vi "固件升级（包含参数恢复）.vi"() -> (3 "结果字符串":string)   [LabVIEW 2016, in "斯坦道总磷总氮.lvlib"]
uses:
  <vilib>/NI/Progress Bar/Controls/Progress Bar Properties.ctl
  <vilib>/Utility/error.llb/DialogType.ctl
  <vilib>/NI/Progress Bar/Progress Bar.lvlib
panel:
  out "布尔":bool
  out "仪器公式":T1(array[cluster])
  out "量程参数":T2(array[cluster])
  out "试剂容量参数":T3
  out "外设参数":cluster{"仪器版本":T4, "error out":errorcluster}
  out "固件升级步骤":T5
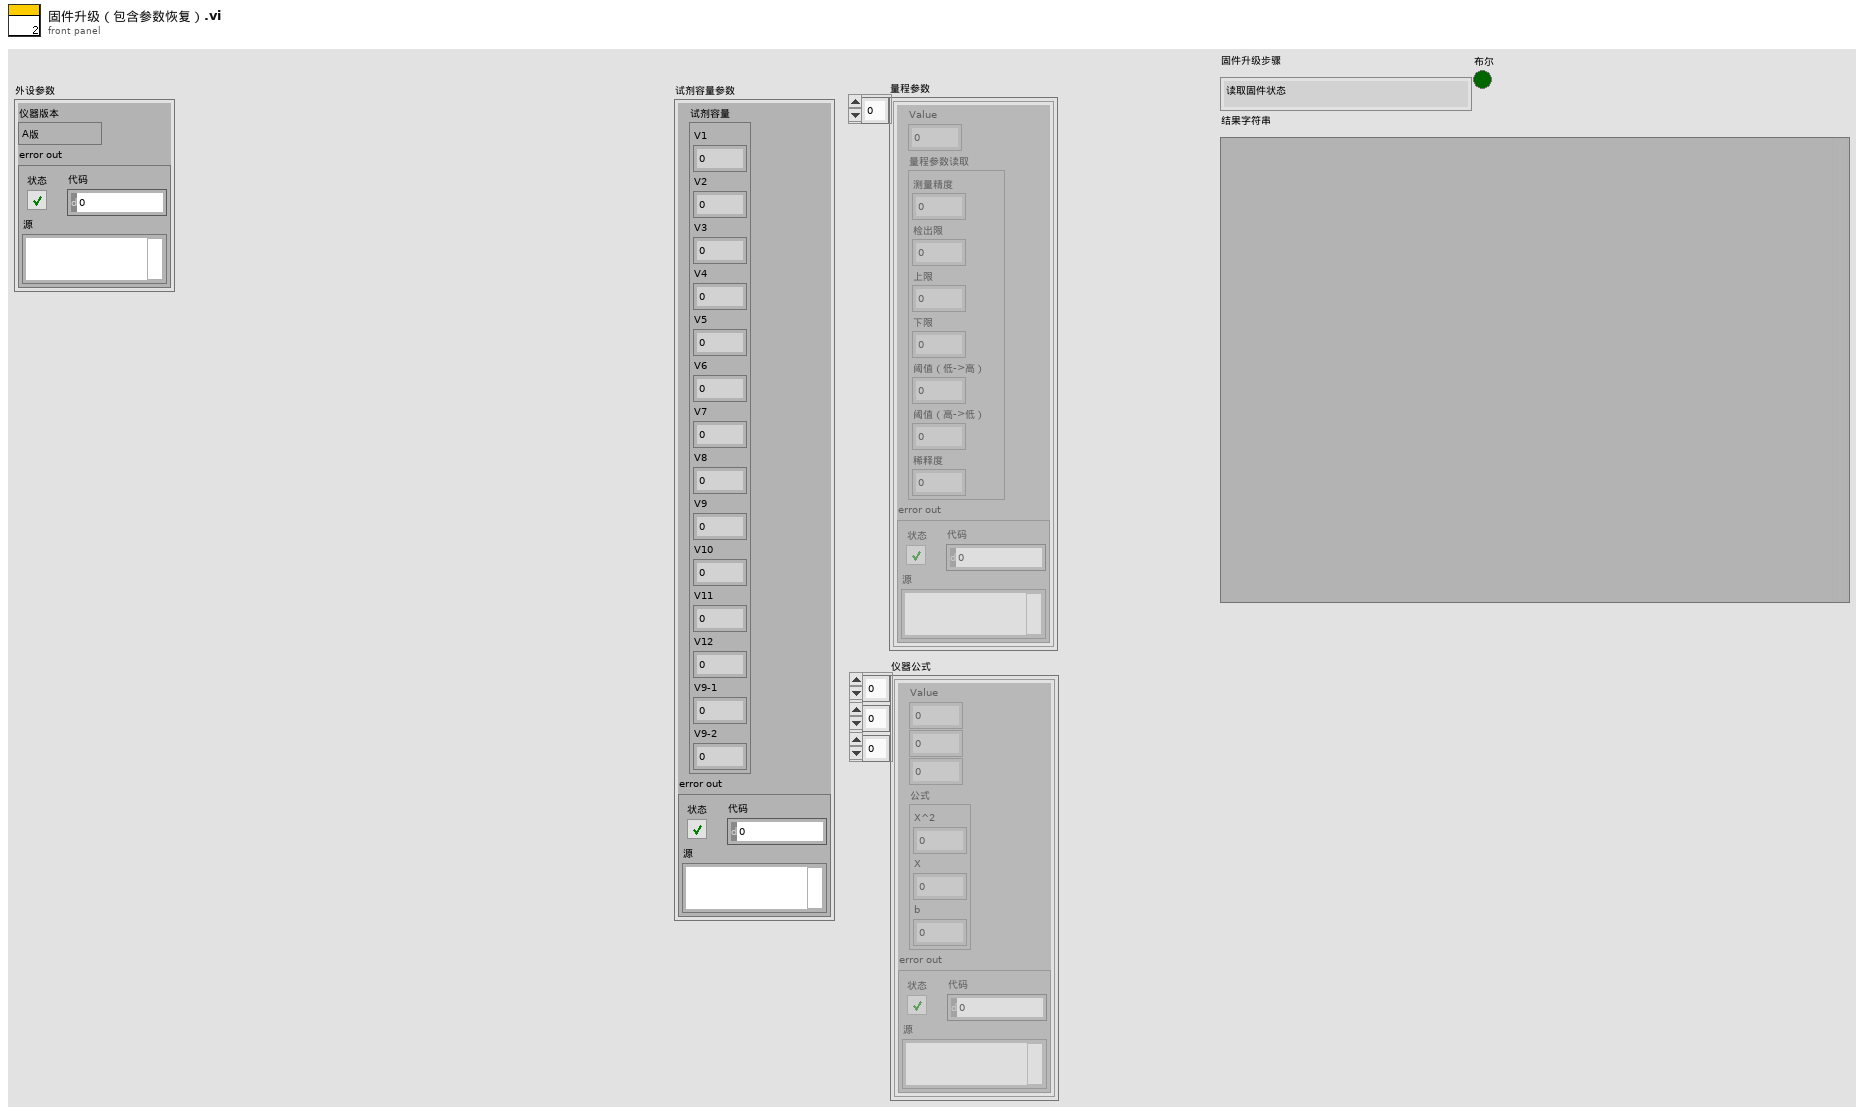
[diagram p1: front panel]
types:
  T1 = cluster{"Value":u16, i32, i32, "公式":cluster{"X^2":dbl, "X":dbl, "b":dbl}, "error out":errorcluster}[][][]
  T2 = cluster{"Value":u16, "量程参数读取":cluster{"测量精度":u16, "检出限":dbl, "上限":dbl, "下限":dbl, "阈值（低->高）":dbl, "阈值（高->低）":dbl, "稀释度":dbl}, "error out":errorcluster}[]
  T3 = cluster{"试剂容量":cluster{"V1":sgl, "V2":sgl, "V3":sgl, "V4":sgl, "V5":sgl, "V6":sgl, "V7":sgl, "V8":sgl, "V9":sgl, "V10":sgl, "V11":sgl, "V12":sgl, "V9-1":sgl, "V9-2":sgl}, "error out":errorcluster}
  T4 = typedef "SingleStepTestV3.lvlib/SingleStepTestV3.lvclass/仪器版本.ctl" = enum16{"A版", "B版", "A1版"}
  T5 = typedef "斯坦道总磷总氮.lvlib/固件升级步骤.ctl" = enum16{"读取固件状态", "备份参数", "写入仪器固件", "恢复参数", "询问是否写入流程", "写入测试流程", "结束"}
  T6 = typedef "Progress Bar.lvlib/Progress Bar Properties.ctl" = cluster{"Background Color":u32, "Installer Title":string, "Title Color":u32, "Action Text":string, "Text Color":u32, "Slider Value":u8, "Bar Color":u32, "Timeout":i32}
  T7 = typedef "DialogType.ctl" = u16
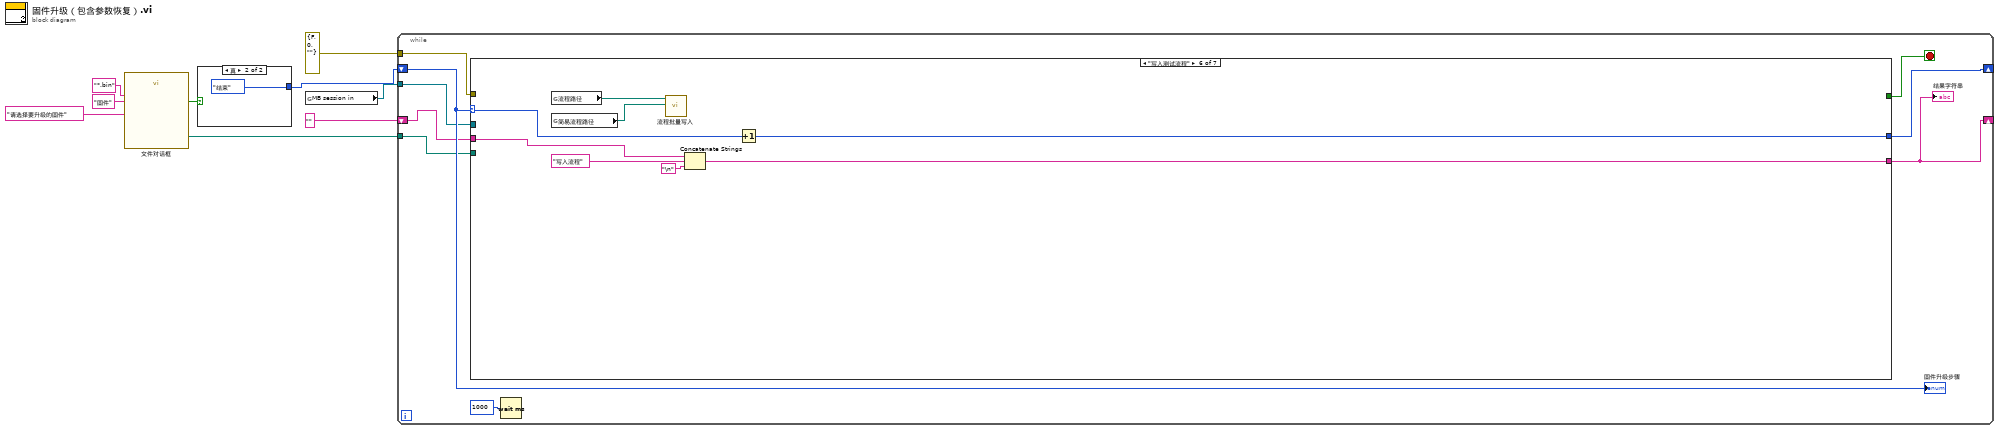
[diagram p0: block diagram]
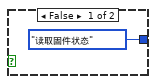
[diagram p2: hidden frame]
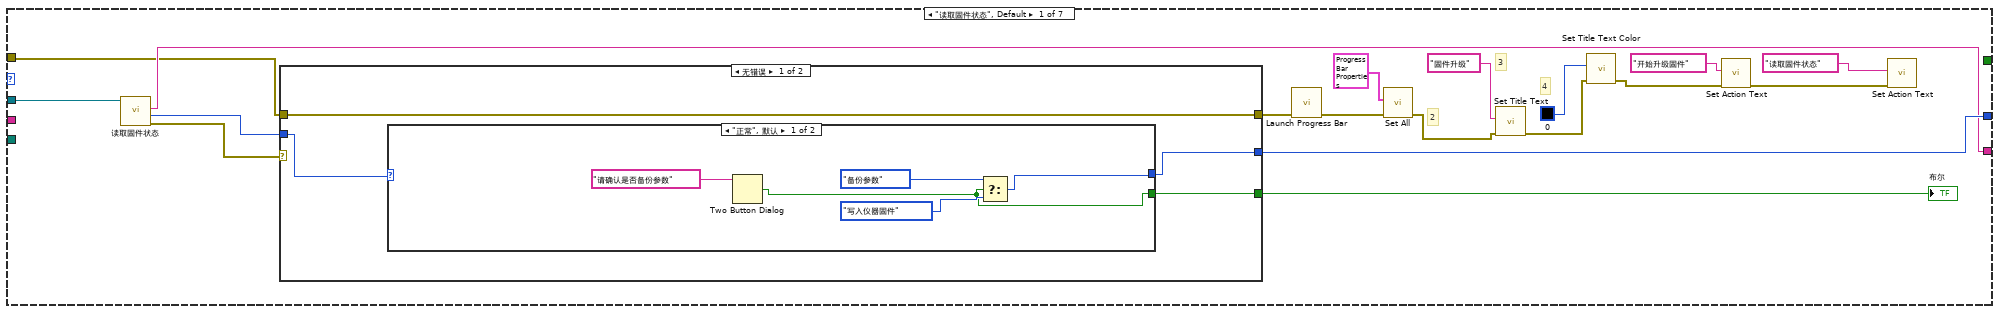
[diagram p3: hidden frame]
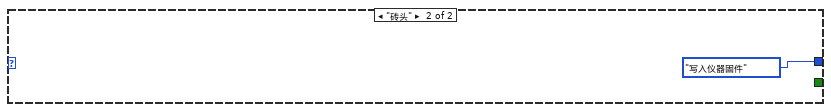
[diagram p4: hidden frame]
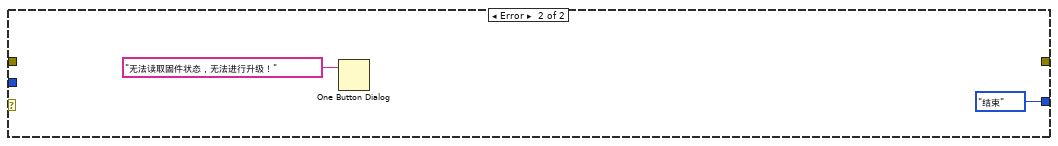
[diagram p5: hidden frame]
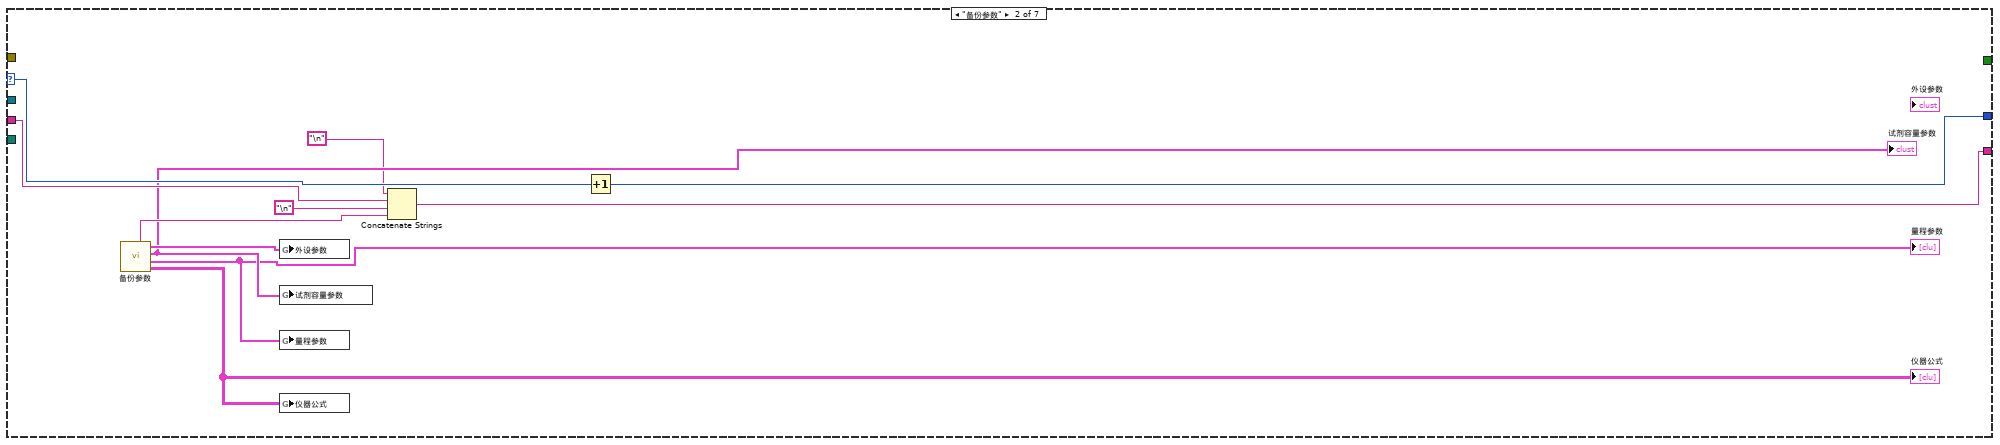
[diagram p6: hidden frame]
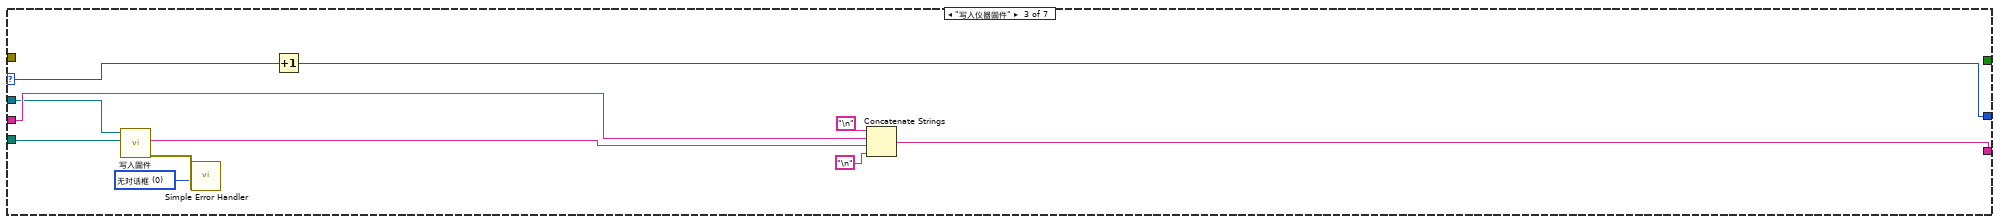
[diagram p7: hidden frame]
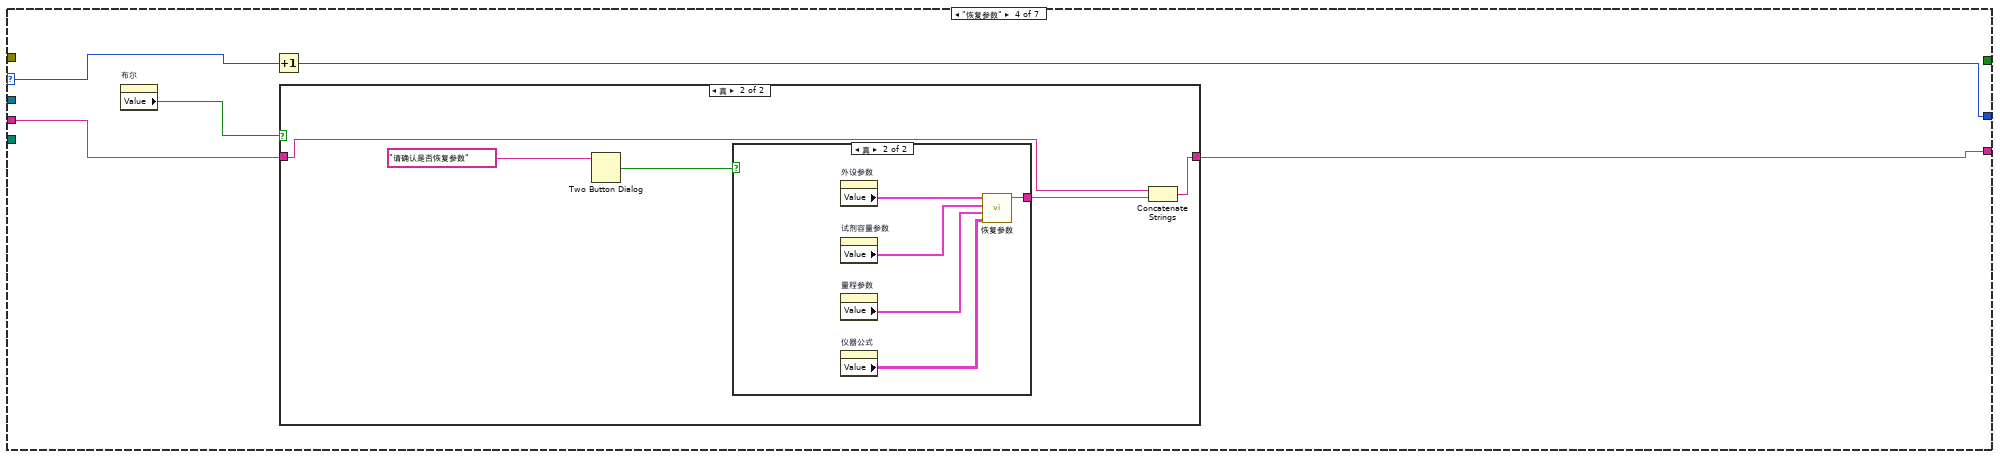
[diagram p8: hidden frame]
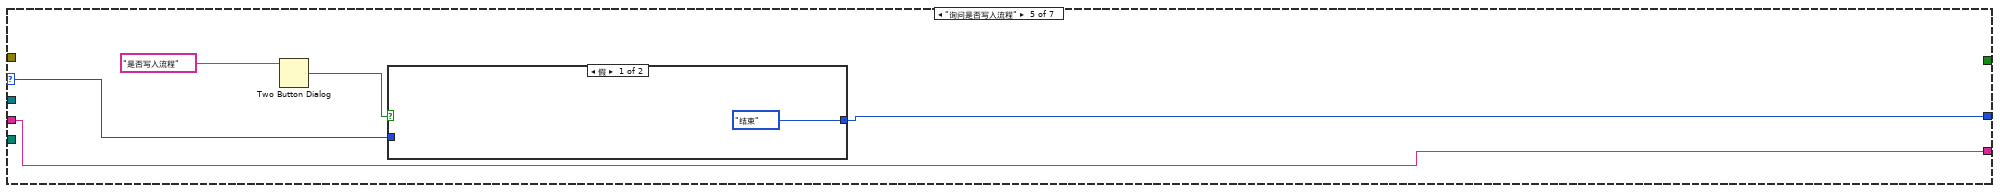
[diagram p11: hidden frame]
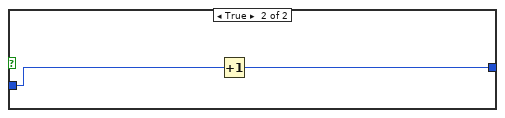
[diagram p12: hidden frame]
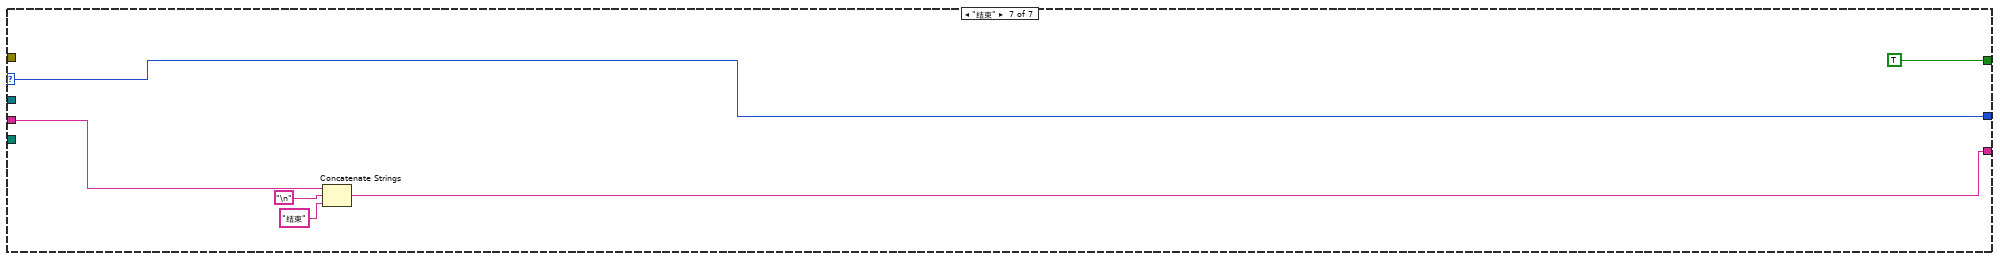
[diagram p13: hidden frame]
diagram:
  n1 = call "文件对话框"("prompt"="请选择要升级的固件", "pattern (all files)"="*.bin", "pattern label"="固件") -> ("selected path"=w4:path, "cancelled"=w2:bool)  [unwired: 9 in, 2 out]
  n2 = case shown="真" w2 {
    tunnel: [固件升级步骤."读取固件状态" ("固件升级步骤") 固件升级步骤."结束" ("固件升级步骤")] -> w3
    frame False {
    }
    frame True {
    }
  }
  n3 = global read "VAR总磷总氮全局变量.vi" "MB session in"() -> (w9:refnum<class "MB_Master.lvclass">)
  n4 = while {
    tunnel: w9 -> [w19]
    shift-right: [w18] -> _
    shift-left: w3 -> [w20]
    shift-right: [w14] -> _
    shift-left: "" ("结果字符串") -> [w15]
    tunnel: w4 -> [w13]
    tunnel: errorcluster {"status"=FALSE, "code"=0, "source"=""} ("error out") -> [w12]
    stop <- w17 stop-if-true
    n5 = case shown="\"写入测试流程\"" w20 {
      selector: w20 -> [_ w61 w72 w74 w91 w102 w109]
      tunnel: w19 -> [w38 _ w68 _ _ _ _]
      tunnel: [w35 w60 w71 w73 w90 w101 w109] -> w18
      tunnel: [_ _ _ _ _ _ TRUE] -> w17
      tunnel: [w34 w59 w69 w76 w89 w99 w105] -> w14
      tunnel: w15 -> [_ w58 w70 w77 w89 w100 w106]
      tunnel: w12 -> [w22 _ _ _ _ _ _]
      tunnel: w13 -> [_ _ w67 _ _ _ _]
      frame "读取固件状态", Default {
        # "4"
        # "3"
        # "2"
        n6 = call "读取固件状态.vi"("MB session in"=w38) -> ("error out"=w36:errorcluster, "固件状态"=w37:enum16{"正常", "砖头"}, "结果字符串"=w34:string)  [unwired: 7 in, 1 out]
        n7 = case shown="无错误" w36 {
          tunnel: w37 -> [w42 _]
          tunnel: [w41 固件升级步骤."结束" ("固件升级步骤")] -> w35
          tunnel: [w40 _] -> w32
          tunnel: w22 -> [w39 _]
          tunnel: [w39 _] -> w21
          frame No Error {
            n8 = case shown="\"正常\", 默认" w42 {
              tunnel: [w43 固件升级步骤."写入仪器固件" ("固件升级步骤")] -> w41
              tunnel: [w44 _] -> w40
              frame "正常", Default {
                n9 = Two Button Dialog(message="请确认是否备份参数" ("消息")) -> (T button?=w44:bool)  [unwired: 2 in]
                n10 = Select(t=固件升级步骤."备份参数" ("固件升级步骤"), s=w44, f=固件升级步骤."写入仪器固件" ("固件升级步骤")) -> (s? t:f=w43:T5)
              }
              frame "砖头" {
              }
            }
          }
          frame Error {
            n11 = One Button Dialog(message="无法读取固件状态，无法进行升级！" ("消息")) -> ()  [unwired: 1 in, 1 out]
          }
        }
        "布尔" <- w32
        n12 = call <vilib>:"Launch Progress Bar.vi"("error in (no error)"=w21) -> ("error out"=w29:errorcluster)  [unwired: 9 in, 1 out]
        n13 = call <vilib>:"Set All.vi"("error in (no error)"=w29, "Progress Bar Properties (Default)"=T6 {"Background Color"=3381759, "Installer Title"="Progress", "Title Color"=0, "Action Text"="", "Text Color"=0, "Slider Value"=0, "Bar Color"=6618880, "Timeout"=30000} ("Progress Bar Properties")) -> ("error out"=w26:errorcluster)  [unwired: 9 in]
        n14 = call <vilib>:"Set Title Text.vi"("error in (no error)"=w26, "Installer Title"="固件升级") -> ("error out"=w24:errorcluster)  [unwired: 9 in]
        n15 = call <vilib>:"Set Title Text Color.vi"("error in (no error)"=w24, "Color Box"=u32 0) -> ("error out"=w27:errorcluster)  [unwired: 9 in]
        n16 = call <vilib>:"Set Action Text.vi"("error in (no error)"=w27, "Action Text"="开始升级固件") -> ("error out"=w31:errorcluster)  [unwired: 9 in]
        n17 = call <vilib>:"Set Action Text.vi"("error in (no error)"=w31, "Action Text"="读取固件状态") -> ()  [unwired: 9 in, 1 out]
      }
      frame "备份参数" {
        n18 = call "备份参数.vi"() -> ("仪器公式"=w52:T1, "量程参数"=w53:T2, "试剂容量参数"=w54:T3, "外设参数"=w55:cluster{"仪器版本":T4, "error out":errorcluster}, "备份结果"=w56:string)  [unwired: 7 in]
        "试剂容量参数" <- w54
        "量程参数" <- w53
        "仪器公式" <- w52
        n19 = global write "VAR总磷总氮全局变量.vi" "外设参数"(w55) -> ()
        n20 = global write "VAR总磷总氮全局变量.vi" "试剂容量参数"(w54) -> ()
        n21 = global write "VAR总磷总氮全局变量.vi" "量程参数"(w53) -> ()
        n22 = global write "VAR总磷总氮全局变量.vi" "仪器公式"(w52) -> ()
        n23 = Concatenate Strings("\n", w58, "\n", w56) -> (w59:string)
        n24 = Increment(x=w61) -> (x+1=w60:T5)
      }
      frame "写入仪器固件" {
        w63 = T7 0 items=["无对话框", "确定信息", "继续或停止信息", "确定信息＋警告", "继续/停止+警告"] ("type of dialog (OK msg:1)")
        n25 = call "写入固件.vi"("selected path"=w67, "MB session in"=w68) -> ("error out"=w64:errorcluster, "结果字符串"=w65:string)  [unwired: 7 in, 1 out]
        n26 = call <vilib>:"Simple Error Handler.vi"("type of dialog (OK msg:1)"=w63, "error in (no error)"=w64) -> ()  [unwired: 3 in, 5 out]
        n27 = Increment(x=w72) -> (x+1=w71:T5)
        n28 = Concatenate Strings("\n", w70, w65, "\n") -> (w69:string)
      }
      frame "恢复参数" {
        n29 = property on="布尔" class="Bool (严格)"() -> ("Value"=w75:bool)  [unwired: 2 in, 2 out]
        n30 = Increment(x=w74) -> (x+1=w73:T5)
        n31 = case shown="真" w75 {
          tunnel: w77 -> [w78 w82]
          tunnel: [w78 w81] -> w76
          frame False {
          }
          frame True {
            n32 = Two Button Dialog(message="请确认是否恢复参数" ("消息")) -> (T button?=w79:bool)  [unwired: 2 in]
            n33 = case shown="真" w79 {
              tunnel: [_ w84] -> w83
              frame False {
              }
              frame True {
                n34 = property on="外设参数" class="Clust (严格)"() -> ("Value"=w88:cluster{"仪器版本":T4, "error out":errorcluster})  [unwired: 2 in, 2 out]
                n35 = property on="试剂容量参数" class="Clust (严格)"() -> ("Value"=w87:T3)  [unwired: 2 in, 2 out]
                n36 = property on="量程参数" class="Arr (严格)"() -> ("Value"=w86:T2)  [unwired: 2 in, 2 out]
                n37 = property on="仪器公式" class="Arr (严格)"() -> ("Value"=w85:T1)  [unwired: 2 in, 2 out]
                n38 = call "恢复参数.vi"("仪器公式"=w85, "量程参数"=w86, "试剂容量参数"=w87, "外设参数"=w88) -> ("恢复结果"=w84:string)  [unwired: 7 in]
              }
            }
            n39 = Concatenate Strings(w82, w83) -> (w81:string)
          }
        }
      }
      frame "询问是否写入流程" {
        n40 = Two Button Dialog(message="是否写入流程" ("消息")) -> (T button?=w92:bool)  [unwired: 2 in]
        n41 = case shown="假" w92 {
          tunnel: w91 -> [_ w96]
          tunnel: [固件升级步骤."结束" w95] -> w90
          frame False {
          }
          frame True {
            n42 = Increment(x=w96) -> (x+1=w95:T5)
          }
        }
      }
      frame "写入测试流程" {
        n43 = global read "总磷总氮断电保存全局变量.vi" "流程路径"() -> (w104:path)
        n44 = global read "总磷总氮断电保存全局变量.vi" "简易流程路径"() -> (w103:path)
        n45 = call "流程批量写入.vi"("简易流程路径"=w103, "添加的路径"=w104) -> ()  [unwired: 10 in]
        n46 = Concatenate Strings(w100, "写入流程" ("字符串"), "\n") -> (w99:string)
        n47 = Increment(x=w102) -> (x+1=w101:T5)
      }
      frame "结束" {
        n48 = Concatenate Strings(w106, "\n", "结束" ("字符串")) -> (w105:string)
      }
    }
    "结果字符串" <- w14
    n49 = Wait (ms)(milliseconds to wait=u32 1000 ("等待时间（毫秒）")) -> ()  [unwired: 1 out]
    "固件升级步骤" <- w20
  }
